vi "dfd_nMAC_CircAddONEwEn.vi"(1 "len":fxp<+,16,16>, 2 "idxIn":fxp<+,16,16>, 3 "Enable":bool) -> (6 "wrap?":bool, 7 "idxOut":fxp<+,16,16>)   [LabVIEW 2017]
doc: "wrap? is cleared if Enable==False."
uses:
  <vilib>/rvi/FXPMathLib/basic elements/FxpAddSub/XNode/nifxpmath_AddSub.xnode
  <vilib>/rvi/FXPMathLib/sim/FxpSim.dll
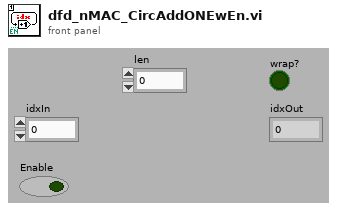
[diagram p1: front panel]
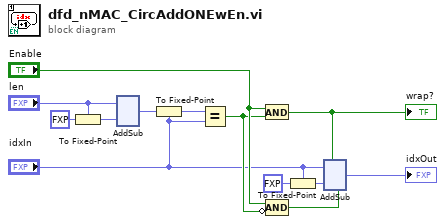
[diagram p0: block diagram]
diagram:
  n1 = To Fixed-Point(fixed-point type="len", number=fxp<+,1,1> 1.0 ("y")) -> (fixed-point=w5:fxp<+,16,16>)
  n2 = xnode "AddSub"("x"="len", "y"=w5) -> ("s"=w6:fxp<+,16,16>)  [unwired: 1 out]
  n3 = To Fixed-Point(fixed-point type="idxIn", number=w6) -> (fixed-point=w3:fxp<+,16,16>)
  n4 = Equal?(x=w3, y="idxIn") -> (x = y?=w9:bool)
  n5 = And(x="Enable", y=w9) -> (x .and. y?=w11:bool)
  "wrap?" <- w11
  n6 = Compound Arithmetic op=AND("Enable", invert w9) -> (w8:bool)
  n7 = To Fixed-Point(fixed-point type="idxIn", number=fxp<+,1,1> 0.0 ("step")) -> (fixed-point=w2:fxp<+,16,16>)
  n8 = xnode "AddSub"("x"="idxIn", "y"=w2, "carry-in"=w8, "use zero instead of x"=w11) -> ("s"=→"idxOut":fxp<+,16,16>)  [unwired: 1 out]
